vi "testCode_planecovertion.vi"() -> ()   [LabVIEW 2020]
panel:
  in  "ArbitraryPlaneStop":T1
  out "StopNormalised":dbl[][](array[numeric])
  out "StartNormalised":dbl[][](array[numeric])
  in  "FrameSize":i32
  in  "ArbitraryPlaneStart":T1
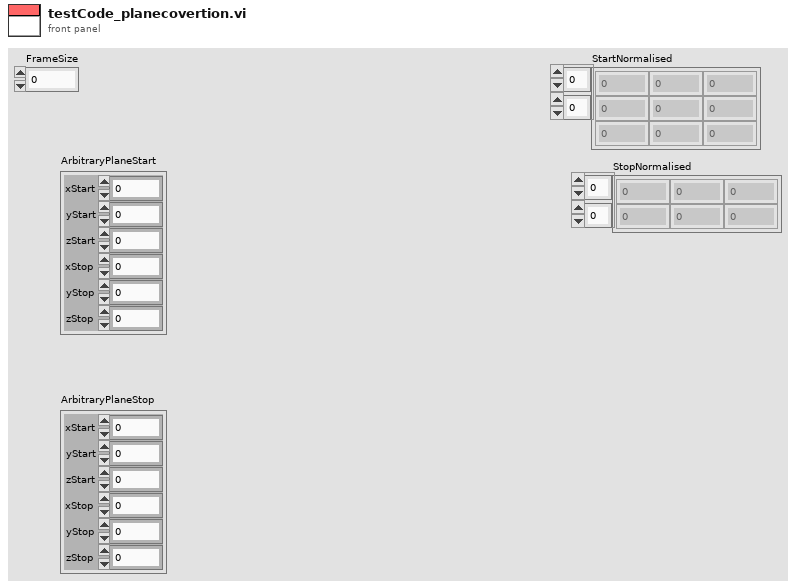
[diagram p1: front panel]
types:
  T1 = cluster{"xStart":dbl, "yStart":dbl, "zStart":dbl, "xStop":dbl, "yStop":dbl, "zStop":dbl}
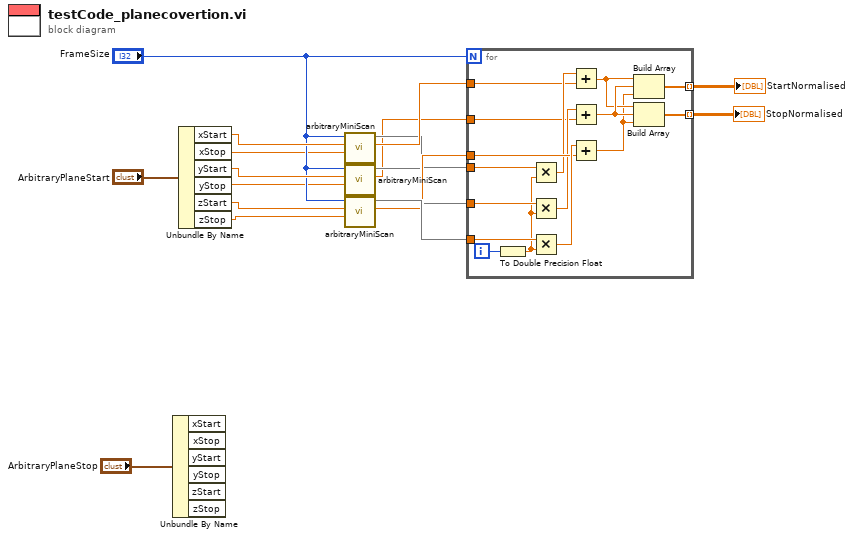
[diagram p0: block diagram]
diagram:
  n1 = Unbundle By Name("ArbitraryPlaneStop") -> ()  [unwired: 6 out]
  n2 = Unbundle By Name("ArbitraryPlaneStart") -> ("xStart"=w10:dbl, "xStop"=w3:dbl, "yStart"=w11:dbl, "yStop"=w2:dbl, "zStart"=w15:dbl, "zStop"=w1:dbl)
  n3 = call "arbitraryMiniScan.vi"("Norm zStop in"=w3, "Norm zStart"=w10, "FrameSize"="FrameSize") -> ("min_coordinate"=w8:dbl, 3:w7)  [unwired: 6 in, 1 out]
  n4 = call "arbitraryMiniScan.vi"("Norm zStop in"=w2, "Norm zStart"=w11, "FrameSize"="FrameSize") -> ("min_coordinate"=w5:dbl, 3:w6)  [unwired: 6 in, 1 out]
  n5 = call "arbitraryMiniScan.vi"("Norm zStop in"=w1, "Norm zStart"=w15, "FrameSize"="FrameSize") -> ("min_coordinate"=w14:dbl, 3:w16)  [unwired: 6 in, 1 out]
  n6 = for {
    N: "FrameSize" -> [_]
    tunnel: [w33] -> w13 mode=indexing
    tunnel: [w32] -> w12 mode=indexing
    tunnel: w16 -> [w30]
    tunnel: w14 -> [w28]
    tunnel: w8 -> [w23]
    tunnel: w7 -> [w19]
    tunnel: w6 -> [w22]
    tunnel: w5 -> [w21]
    i -> [w31]
    n7 = To Double Precision Float(number=w31) -> (double precision float=w20:dbl)
    n8 = Multiply(x=w19, y=w20) -> (x*y=w26:dbl)
    n9 = Multiply(x=w22, y=w20) -> (x*y=w27:dbl)
    n10 = Multiply(x=w30, y=w20) -> (x*y=w29:dbl)
    n11 = Add(x=w26, y=w23) -> (x+y=w24:dbl)
    n12 = Add(x=w27, y=w21) -> (x+y=w25:dbl)
    n13 = Add(x=w29, y=w28) -> (x+y=w18:dbl)
    n14 = Build Array(w24, w25, w18) -> (w33:dbl[])
    n15 = Build Array(w24, w25, w18) -> (w32:dbl[])
  }
  "StartNormalised" <- w13
  "StopNormalised" <- w12
